vi "FT_Reset_Device.vi"(8 "error in (no error)":errorcluster, 11 "Handle In":u64) -> (0 "error out":errorcluster, 1 "FT_Status":u32(ring) items=["FT_OK", "FT_INVALID_HANDLE", "FT_DEVICE_NOT_FOUND", "FT_DEVICE_NOT_OPENED", "FT_IO_ERROR", "FT_INSUFFICIENT_RESOURCES", "FT_INVALID_PARAMETER", "FT_INVALID_BAUD_RATE", "FT_DEVICE_NOT_OPENED_FOR_ERASE", "FT_DEVICE_NOT_OPENED_FOR_WRITE", "FT_FAILED_TO_WRITE_DEVICE", "FT_EEPROM_READ_FAILED", "FT_EEPROM_WRITE_FAILED", "FT_EEPROM_ERASE_FAILED", "FT_EEPROM_NOT_PRESENT", "FT_EEPROM_NOT_PROGRAMMED", "FT_INVALID_ARGS", "FT_NOT_SUPPORTED", "FT_OTHER_ERROR"], 3 "Handle Out":u64)   [LabVIEW 2020]
uses:
  FTD2XX.dll
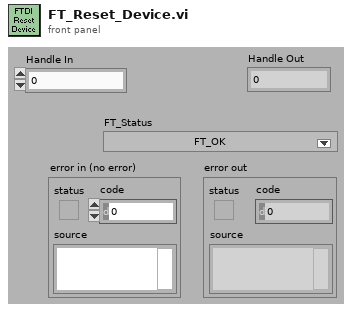
[diagram p1: front panel]
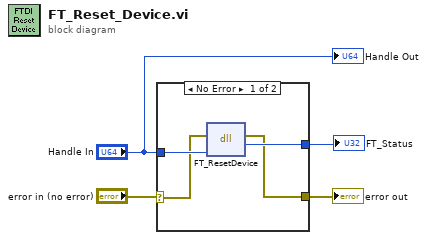
[diagram p0: block diagram]
diagram:
  n1 = case shown="No Error" "error in (no error)" {
    selector: "error in (no error)" -> [w6 w9]
    tunnel: "Handle In" -> [w8 _]
    tunnel: [w7 _] -> w4
    tunnel: [w5 w9] -> w2
    frame No Error {
      n2 = dll-call lib="FTD2XX.dll" fn="FT_ResetDevice"(error in=w6, "Handle"=w8) -> (error out=w5:errorcluster, "FT_Status"=w7:u32)  [unwired: 3 in, 1 out]
    }
    frame Error {
    }
  }
  "FT_Status" <- w4
  "error out" <- w2
  "Handle Out" <- "Handle In"
